vi "zadanie7_3.vi"() -> ()   [LabVIEW 2012]
panel:
  out "krzywe lissajous":cluster{"Y":dbl[], "Y":dbl[]}[](graph)
  in  "reet_signal2":bool
  in  "reet_signal1":bool
  in  "stop":bool
  in  "amplitude 2":dbl
  in  "alfa 2":dbl(knob) scale=0.0..100.0
  in  "amplitude":dbl
  in  "alfa":dbl(knob) scale=0.0..100.0
  out "koło":cluster{"X":dbl, "Y":dbl}[](graph)
  out "zaloguj":bool
  out "haslo":string
  out "login":string
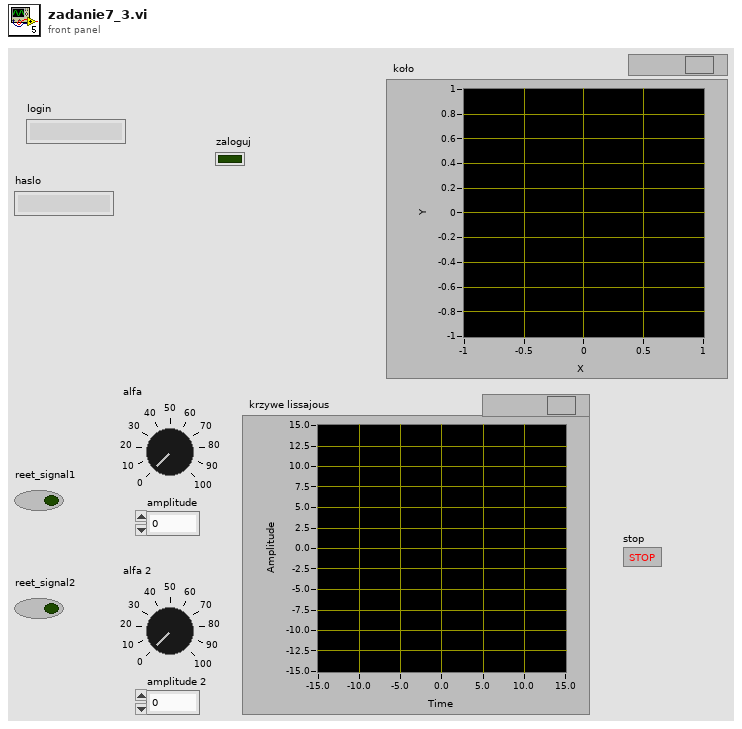
[diagram p1: front panel]
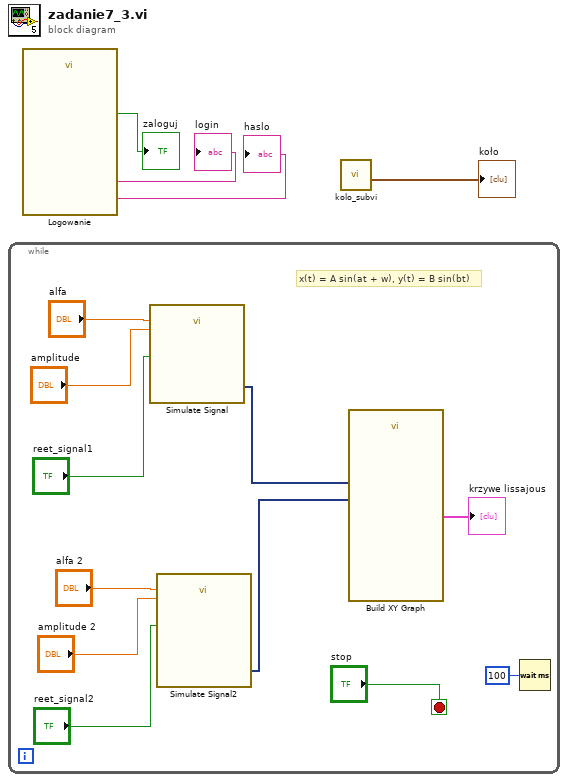
[diagram p0: block diagram]
diagram:
  n1 = while {
    stop <- "stop" stop-if-true
    # "x(t) = A sin(at + w), y(t) = B sin(bt)"
    n2 = call "Simulate Signal"("Reset Signal"="reet_signal1", "Frequency"="alfa", "Amplitude"="amplitude") -> ("Sine one"=w7:dynamicdata)  [unwired: 11 in, 1 out]
    n3 = call "Simulate Signal2"("Reset Signal"="reet_signal2", "Frequency"="alfa 2", "Amplitude"="amplitude 2") -> ("Sine two"=w6:dynamicdata)  [unwired: 11 in, 1 out]
    n4 = call "Build XY Graph"("Y Input"=w6, "X Input"=w7) -> ("XY Graph"=→"krzywe lissajous":cluster{"Y":dbl[], "Y":dbl[]}[])  [unwired: 3 in, 6 out]
    n5 = Wait (ms)(milliseconds to wait=u32 100) -> ()  [unwired: 1 out]
  }
  n6 = call "Logowanie"() -> ("Podaj hasło:"=→"haslo":string, "Podaj nazwę:"=→"login":string, "Dalej"=→"zaloguj":bool)  [unwired: 16 in, 1 out]
  n7 = call "kolo_subvi.vi"() -> ("XY Graph"=→"koło":cluster{"X":dbl, "Y":dbl}[])  [unwired: 11 in]
